vi "Manual Assembly.vi"() -> ()   [LabVIEW 2020]
uses:
  Classes/Routine/Routine Enum.ctl
  Classes/Assembly/Assembly Run.lvclass
  Classes/Workspace/Fixture Enum.ctl
  Classes/Workspace/Fixture.lvclass
  Classes/Controller/Controller.lvclass
  Classes/Routine/Routine.lvclass
panel:
  in  "Update":bool
  in  "Stage":i32(listbox)=-1
  in  "Routine":T1=enum."Dispense on Plate"
  in  "Stop":bool
  in  "Remove":bool
  in  "Add":bool
  in  "Go":bool
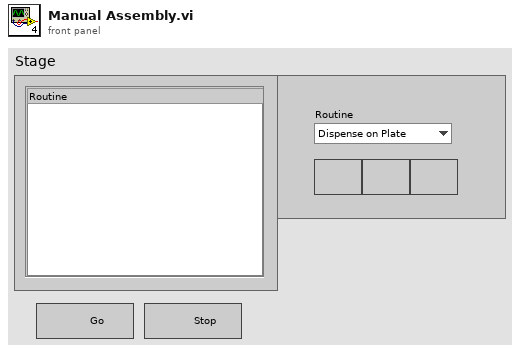
[diagram p1: front panel]
types:
  T1 = typedef "Routine.lvclass/Routine Enum.ctl" = enum16{"Primary Pick Up", "Pick Up All", "Put Down Secondary", "Put Down All", "Release Syringe", "Secondary Pick Up", "Secure Syringe", "Dispense on Plate", "Dispense on Kapton", "Dispense on Sensor"}
  T2 = typedef "Fixture.lvclass/Fixture Enum.ctl" = enum16{"Assembly Tray", "Syringe Space", "Component", "Pick Up Tool", "Current Position"}
  T3 = typedef "Controller.lvclass/Controllers.ctl" = cluster{"I-O.lvclass":refnum<class "I-O.lvclass">, "Dispenser.lvclass":refnum<class "Dispenser.lvclass">, "Gantry":refnum<k24>}
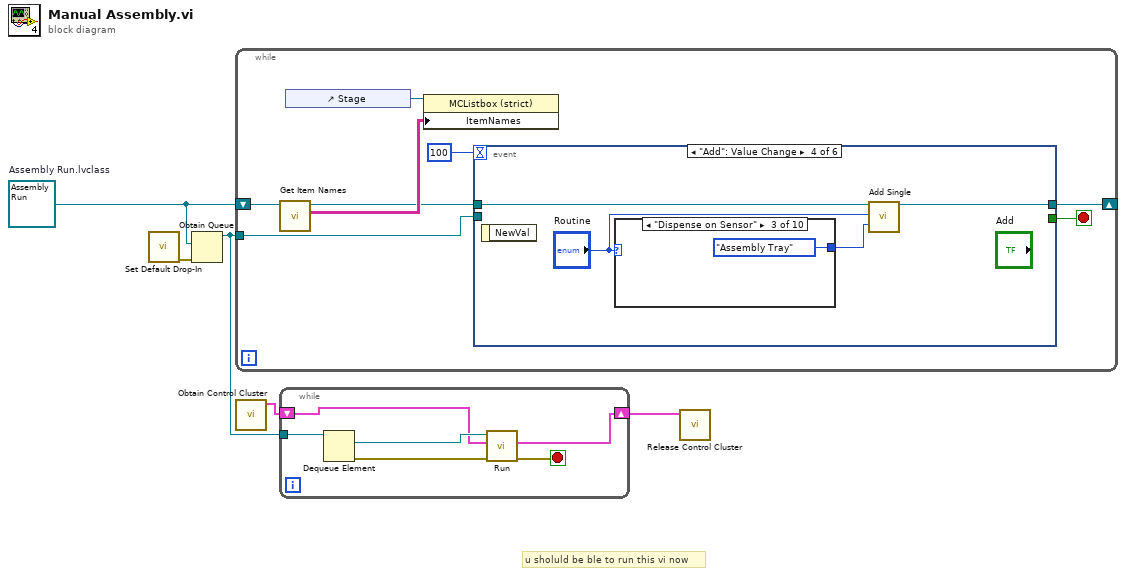
[diagram p0: block diagram]
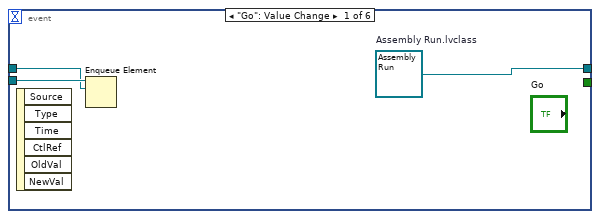
[diagram p2: hidden frame]
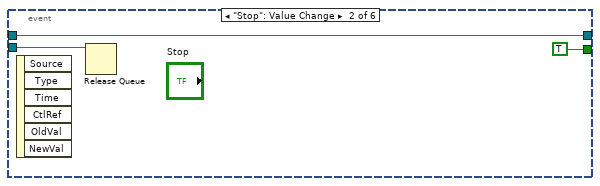
[diagram p3: hidden frame]
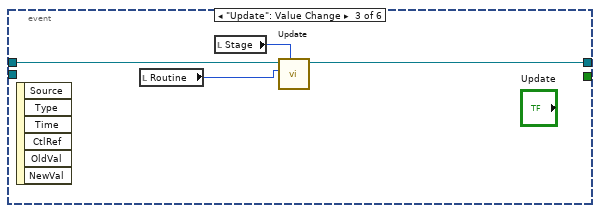
[diagram p4: hidden frame]
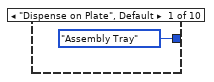
[diagram p5: hidden frame]
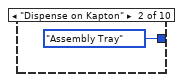
[diagram p6: hidden frame]
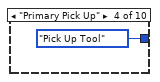
[diagram p7: hidden frame]
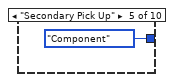
[diagram p8: hidden frame]
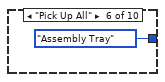
[diagram p9: hidden frame]
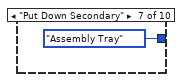
[diagram p10: hidden frame]
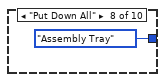
[diagram p11: hidden frame]
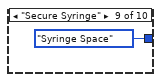
[diagram p12: hidden frame]
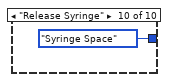
[diagram p13: hidden frame]
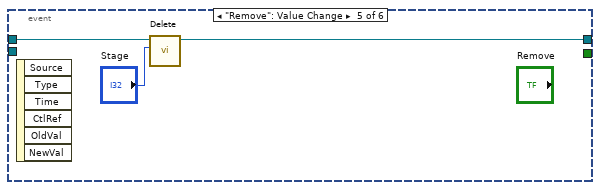
[diagram p14: hidden frame]
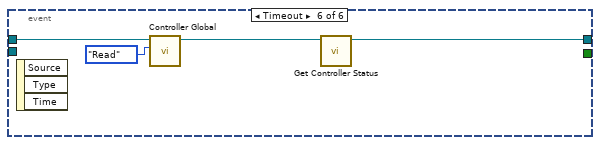
[diagram p15: hidden frame]
diagram:
  w3 = refnum<class "Assembly Run.lvclass"> refnum  # Assembly Run.lvclass
  # "u sholuld be ble to run this vi now"
  n1 = call "Set Default Drop-In.vi"() -> ("error out"=w4:errorcluster)  [unwired: 11 in]
  n2 = Obtain Queue(element data type=w3, error in (no error)=w4) -> (queue out=w5:refnum<queue>)  [unwired: 3 in, 2 out]
  n3 = while {
    shift-right: [w7] -> _
    shift-left: w3 -> [w9]
    tunnel: w5 -> [w12]
    stop <- w13 stop-if-true
    n4 = call "Get Item Names.vi"("Assembly Run in"=w9) -> ("Item names"=w11:string[][], "Assembly Run out"=w8:refnum<class "Assembly Run.lvclass">)  [unwired: 8 in, 1 out]
    n5 = control-ref of="Stage"() -> (w10:refnum<vi>)
    n6 = property class="MCListbox (strict)"(reference=w10, "ItemNames"=w11) -> ()  [unwired: 1 in, 2 out]
    n7 = event shown="[3] \"Add\": Value Change" {
      selector: _ -> [_ _ _ _ _ _]
      dyn-events: _ -> [_ _ _ _ _ _]
      timeout: 100 -> [_ _ _ _ _ _]
      tunnel: [_ TRUE _ _ _ _] -> w13
      tunnel: w8 -> [w15 w18 w23 w27 w40 w44]
      tunnel: [w14 w18 w22 w26 w39 w41] -> w7
      tunnel: w12 -> [w16 w17 _ _ _ _]
      event "Go": Value Change {
        w14 = refnum<class "Assembly Run.lvclass"> refnum  # Assembly Run.lvclass
        n8 = event-data() -> ()  [unwired: 1 in, 6 out]
        n9 = Enqueue Element(queue=w16, element=w15) -> ()  [unwired: 2 in, 3 out]
      }
      event "Stop": Value Change {
        n10 = event-data() -> ()  [unwired: 1 in, 6 out]
        n11 = Release Queue(queue=w17) -> ()  [unwired: 2 in, 3 out]
      }
      event "Update": Value Change {
        n12 = event-data() -> ()  [unwired: 1 in, 6 out]
        n13 = local read "Routine"() -> (w21:T1)
        n14 = local read "Stage"() -> (w20:i32)
        n15 = call "Update.vi"("Row"=w20, "Routine"=w21, "Assembly Run in"=w23) -> ("Assembly Run out"=w22:refnum<class "Assembly Run.lvclass">)  [unwired: 7 in, 1 out]
      }
      event "Add": Value Change {
        n16 = event-data() -> ()  [unwired: 1 in, 1 out]
        n17 = case shown="\"Dispense on Sensor\"" "Routine" {
          tunnel: [Fixture_Enum."Assembly Tray" ("Fixture") Fixture_Enum."Assembly Tray" ("Fixture") Fixture_Enum."Assembly Tray" ("Fixture") Fixture_Enum."Pick Up Tool" ("Fixture") Fixture_Enum."Component" ("Fixture") Fixture_Enum."Assembly Tray" ("Fixture") Fixture_Enum."Assembly Tray" ("Fixture") Fixture_Enum."Assembly Tray" ("Fixture") Fixture_Enum."Syringe Space" ("Fixture") Fixture_Enum."Syringe Space" ("Fixture")] -> w25
          frame "Dispense on Plate", Default {
          }
          frame "Dispense on Kapton" {
          }
          frame "Dispense on Sensor" {
          }
          frame "Primary Pick Up" {
          }
          frame "Secondary Pick Up" {
          }
          frame "Pick Up All" {
          }
          frame "Put Down Secondary" {
          }
          frame "Put Down All" {
          }
          frame "Secure Syringe" {
          }
          frame "Release Syringe" {
          }
        }
        n18 = call-dynamic "Add Single.vi"("UI in"=w27, "Routine"="Routine", "Fixture"=w25) -> ("UI out"=w26:refnum<class "Assembly Run.lvclass">)  [unwired: 15 in, 1 out]
      }
      event "Remove": Value Change {
        n19 = event-data() -> ()  [unwired: 1 in, 6 out]
        n20 = call "Delete.vi"("Index"="Stage", "Assembly In"=w40) -> ("Assembly Out"=w39:refnum<class "Assembly Run.lvclass">)  [unwired: 8 in, 1 out]
      }
      event Timeout {
        n21 = event-data() -> ()  [unwired: 1 in, 3 out]
        n22 = call "Controller Global.vi"("Action"=enum16{"Initialize", "Read", "Write"}."Read", "Assembly Run in"=w44) -> ("Assembly Run out"=w42:refnum<class "Assembly Run.lvclass">)  [unwired: 7 in, 2 out]
        n23 = call "Get Controller Status.vi"("Assembly Run in"=w42) -> ("Assembly Run out"=w41:refnum<class "Assembly Run.lvclass">)  [unwired: 9 in, 1 out]
      }
    }
  }
  n24 = call "Obtain Control Cluster.vi"() -> ("Control Out"=w2:T3)  [unwired: 11 in]
  n25 = while {
    tunnel: w5 -> [w50]
    shift-right: [w45] -> w1
    shift-left: w2 -> [w46]
    stop <- w48 stop-if-true
    n26 = Dequeue Element(queue=w50) -> (element=w47:refnum<class "Assembly Run.lvclass">, error out=w49:errorcluster)  [unwired: 2 in, 2 out]
    n27 = call-dynamic "Run.vi"("error in (no error)"=w49, "Control In"=w46, "Assembly In"=w47) -> ("error out"=w48:errorcluster, "Control Out"=w45:T3)  [unwired: 6 in, 1 out]
  }
  n28 = call "Release Control Cluster.vi"("output cluster"=w1) -> ()  [unwired: 11 in]
